vi "CIMAQ_Create_RGB.vi"   [LabVIEW 2017]
types:
  T1 = typedef "Image Type" = u32
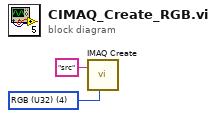
[diagram p0: block diagram]
diagram:
  w1 = T1 4 items=["Grayscale (U8)", "Grayscale (I16)", "Grayscale (SGL)", "Complex (CSG)", "RGB (U32)", "HSL (U32)", "RGB (U64)", "Grayscale (U16)"] ("Image Type")
  n1 = call "IMAQ Create"("Image Name"="src", "Image Type"=w1) -> ()  [unwired: 3 in, 2 out]
